vi "Launch Fault Monitor.vi"(8 "error in (no error)":errorcluster, 11 "Main in":refnum<class "Main.lvclass">) -> (0 "error out":errorcluster, 3 "Main out":refnum<class "Main.lvclass">)   [LabVIEW 2023, in "Main.lvlib" / "Main.lvclass"]
uses:
  Library/Main.lvclass
  builds/Main/Fault Monitor.lvlibp/Library/Fault Monitor.lvclass
  Library/Main.lvclass/Main.ctl
  builds/Framework/Engine.lvlibp/Managed Actor/Library/Managed Actor.lvclass
  builds/Framework/Engine.lvlibp/Engine/Library/Engine.lvclass
  builds/Main/Docking.lvlibp/Docking/Docking.lvclass
  builds/Framework/Panel Manager.lvlibp/Panel/Panel/Subpanel/Subpanel.lvclass
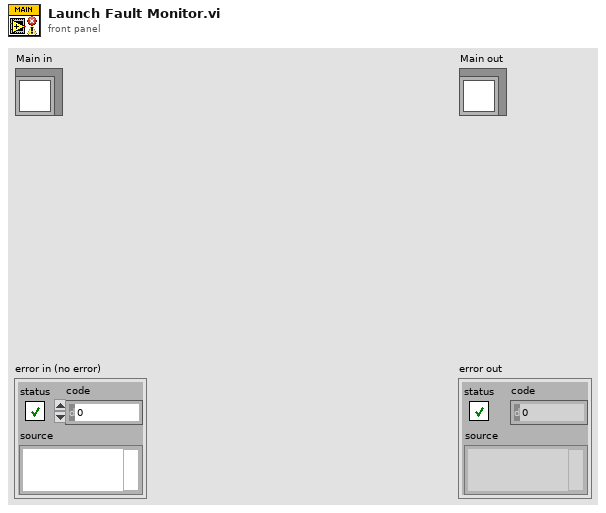
[diagram p1: front panel]
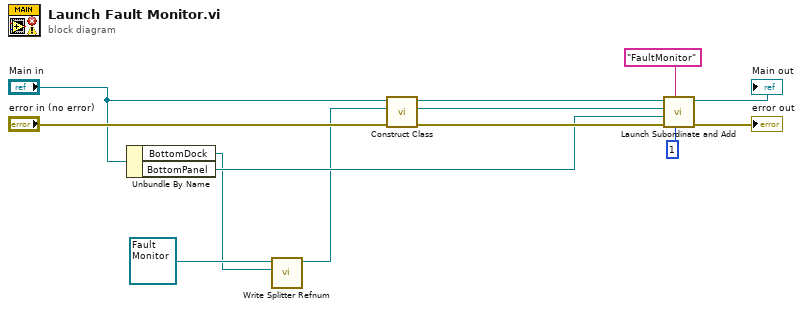
[diagram p0: block diagram]
diagram:
  n1 = Unbundle By Name("Main in") -> ("BottomDock"=w3:refnum<vi>, "BottomPanel"=w6:refnum<class "Subpanel.lvclass">)
  n2 = call "Write Splitter Refnum.vi"("Splitter Refnum"=w3, "Docking in"=refnum<class "Fault Monitor.lvclass"> refnum ("Fault Monitor.lvlibp:Fault Monitor.lvclass")) -> ("Docking out"=w4:refnum<class "Fault Monitor.lvclass">)  [unwired: 8 in, 1 out]
  n3 = call "Construct Class.vi"("error in (no error)"="error in (no error)", "Actor in"=w4, "Engine in"="Main in") -> ("error out"=w10:errorcluster, "Actor out"=w11:refnum<class "Fault Monitor.lvclass">, "Engine out"=w12:refnum<class "Main.lvclass">)  [unwired: 6 in]
  n4 = call "Launch Subordinate and Add.vi"("PanelIndex"=1, "Identifier"="FaultMonitor", "error in (no error)"=w10, "Panel"=w6, "Nested Panel Actor"=w11, "Managed Actor in"=w12) -> ("error out"=→"error out":errorcluster, "Managed Actor out"=→"Main out":refnum<class "Main.lvclass">)  [unwired: 4 in]
